vi "Planet_Meassurement.vi"(8 "error in (no error)":errorcluster, 11 "Conf":T1) -> (0 "error out":errorcluster)   [LabVIEW 2021]
uses:
  Typedefs/Stany.ctl
  Typedefs/Axis.ctl
  Typedefs/OrderAnalysis.ctl
  Typedefs/Start_End.ctl
  Typedefs/PropertiesOrderAnalysis.ctl
  Typedefs/FGV_TDMS.ctl
  Typedefs/GET_SET.ctl
  Typedefs/PropertyUserChange.ctl
  Typedefs/DataToUserInterface.ctl
  Typedefs/MeassurementMode.ctl
  Typedefs/PropertiesRead_TDM.ctl
  <vilib>/DAQmx/create/channels.llb/DAQmx Create Channel (AI-Voltage-Basic).vi
  <vilib>/DAQmx/read.llb/DAQmx Read (Analog 1D Wfm NChan NSamp).vi
  <vilib>/DAQmx/configure/timing.llb/DAQmx Timing (Sample Clock).vi
  Typedefs/Detected peaks.ctl
  Typedefs/All_Queues.ctl
  Typedefs/ConfCluster.ctl
  Typedefs/PlanetInfo.ctl
  Typedefs/AllDataToAnal.ctl
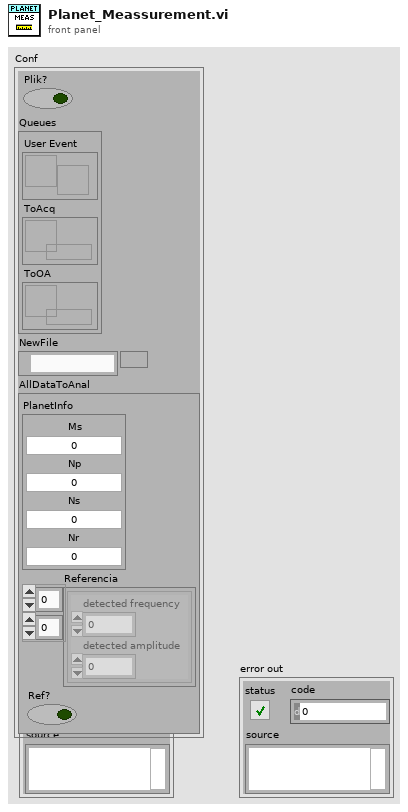
[diagram p1: front panel]
types:
  T1 = typedef "ConfCluster.ctl" = cluster{"Plik?":bool, "Queues":T2, "NewFile":path, "AllDataToAnal":T3}
  T2 = typedef "All_Queues.ctl" = cluster{"User Event":refnum<user-event>, "ToAcq":refnum<queue>, "ToOA":refnum<queue>}
  T3 = typedef "AllDataToAnal.ctl" = cluster{"PlanetInfo":T4, "Referencia":T5[][], "Ref?":bool}
  T4 = typedef "PlanetInfo.ctl" = cluster{"Ms":dbl, "Np":dbl, "Ns":dbl, "Nr":dbl}
  T5 = typedef "Detected peaks.ctl" = cluster{"detected frequency":dbl, "detected amplitude":dbl}
  T6 = typedef "PropertiesRead_TDM.ctl" = cluster{"Start/End":T7, "stop":bool, "file path":path, "OrderAnalysis":T8, "Meassurement Mode":T10}
  T7 = typedef "Start_End.ctl" = enum16{"Start", "End"}
  T8 = typedef "OrderAnalysis.ctl" = cluster{"dB on":bool, "window type":u32, "max order to analyze":dbl, "order resolution":dbl, "Axis":T9, "Sample rate":i64, "Save?":bool, "Multiple_Frequency":i32, "averaging mode":enum16{"No averaging", "Vector averaging", "RMS averaging", "Peak hold"}}
  T9 = typedef "Axis.ctl" = u16
  T10 = typedef "MeassurementMode.ctl" = cluster{"Sample mode":i32, "Terminal conf":i32, "Channels":tag}
  T11 = typedef "Stany.ctl" = enum16{"Idle", "Init", "Acq", "End"}
  T12 = typedef "PropertiesOrderAnalysis.ctl" = cluster{"Start/End":T7, "data":waveform(dbl)[], "OrderAnalysis":T8, "Tacho":waveform(dbl)[]}
  T13 = typedef "PropertyUserChange.ctl" = enum16{"Default", "Results", "Start", "Save", "CanalNames"}
  T14 = typedef "DataToUserInterface.ctl" = cluster{"Value":variant, "Property":T13}
  T15 = typedef "GET_SET.ctl" = enum16{"SET", "GET"}
  T16 = typedef "FGV_TDMS.ctl" = cluster{"Counter":i32, "Syg_GroupName":string, "Syg_ChannelNames":string[], "Tacho_GroupName":string, "Tacho_ChannelNames":string[]}
  T17 = enum16{"open", "open or create", "create or replace", "create", "open (read-only)"}
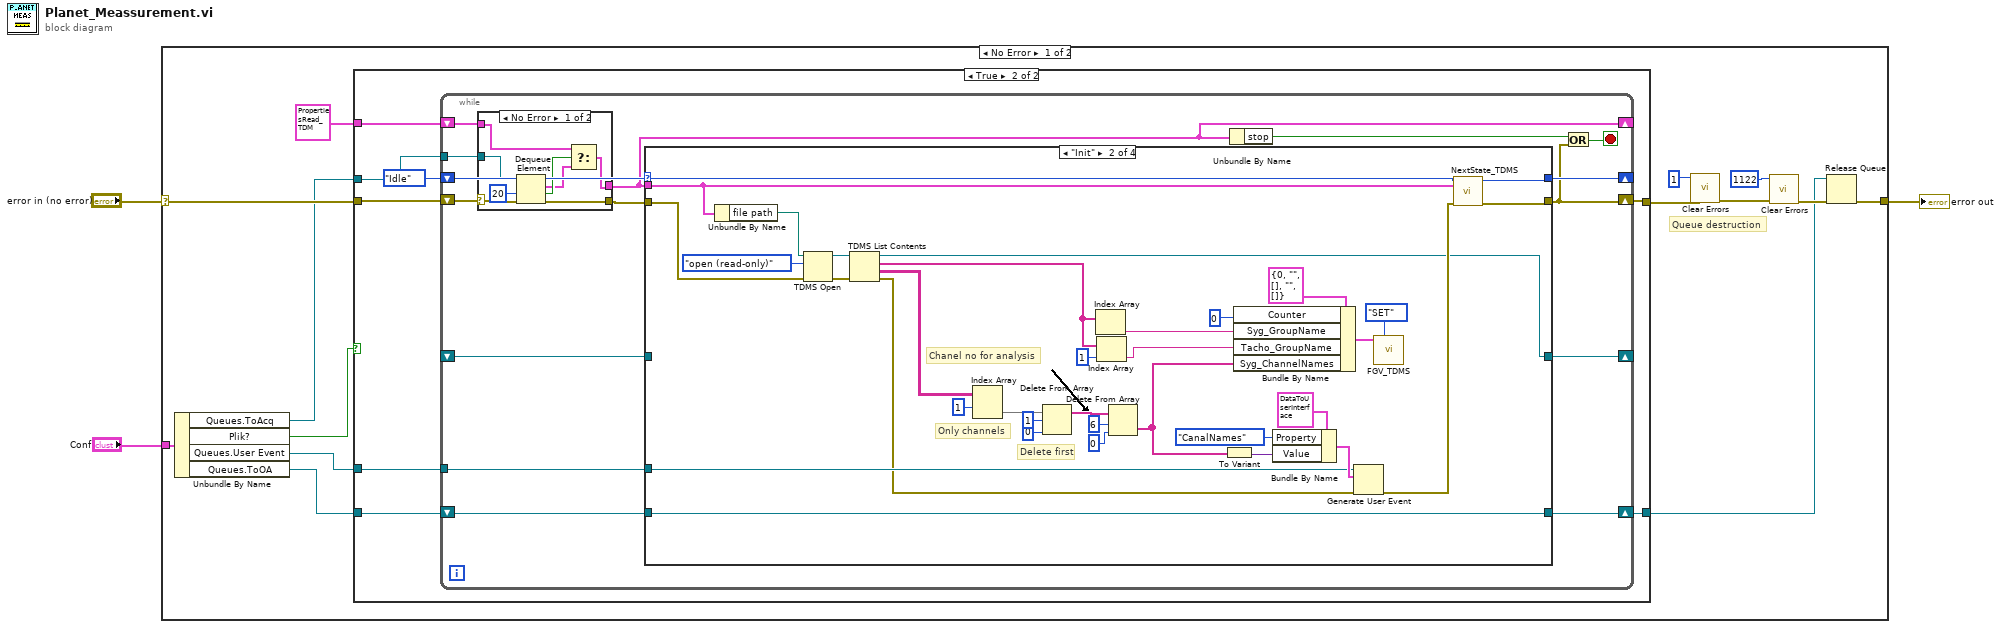
[diagram p0: block diagram]
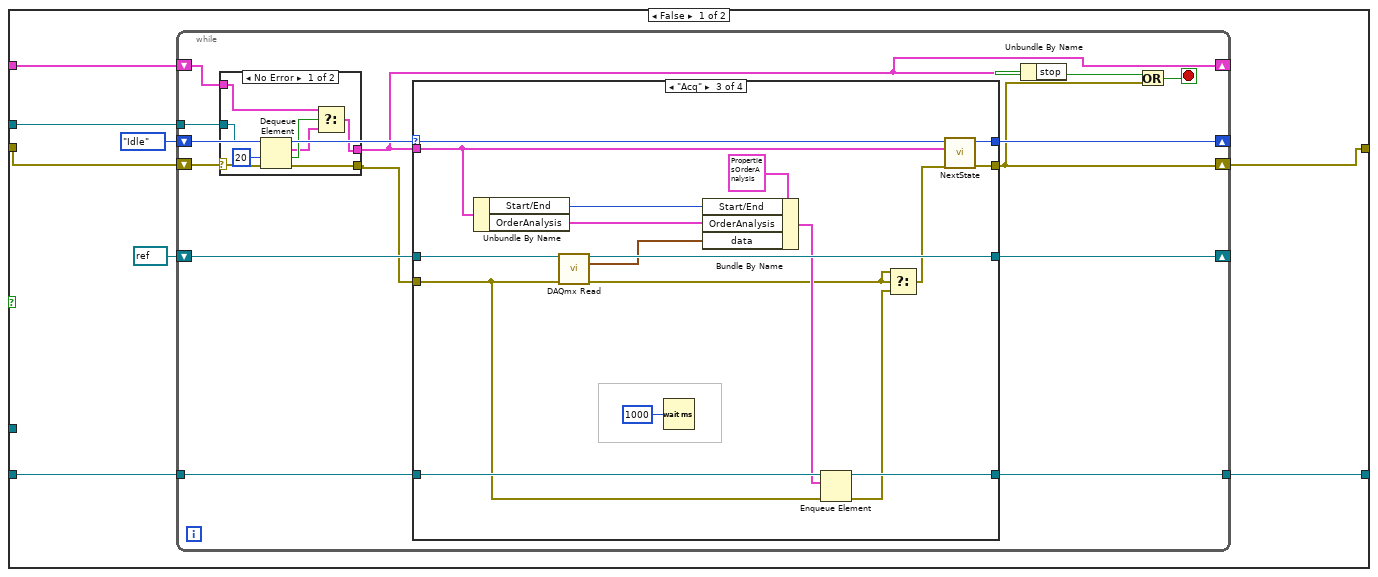
[diagram p2: hidden frame]
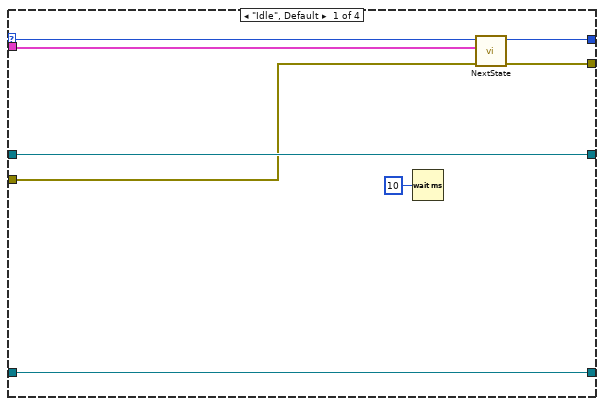
[diagram p4: hidden frame]
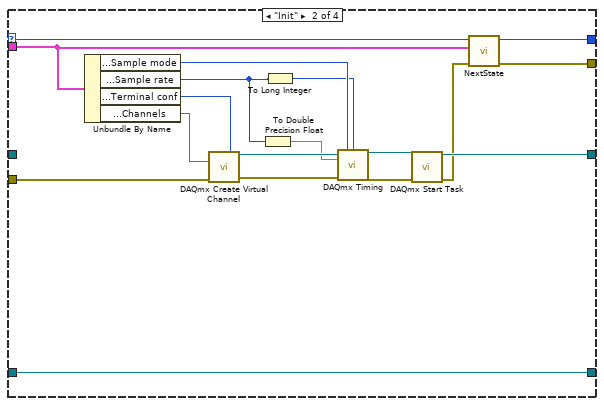
[diagram p5: hidden frame]
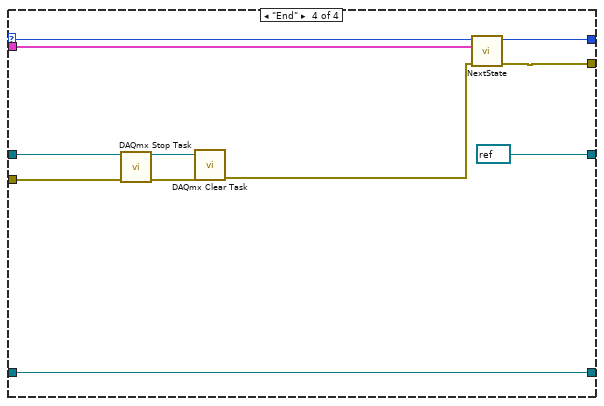
[diagram p6: hidden frame]
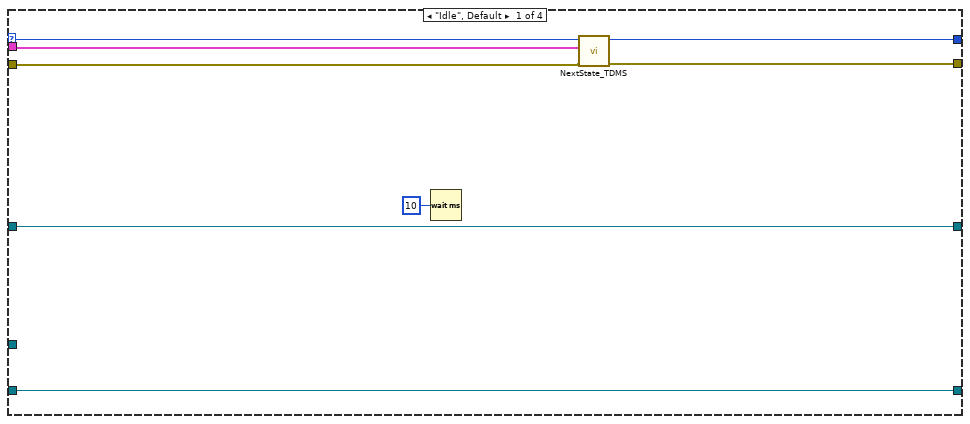
[diagram p8: hidden frame]
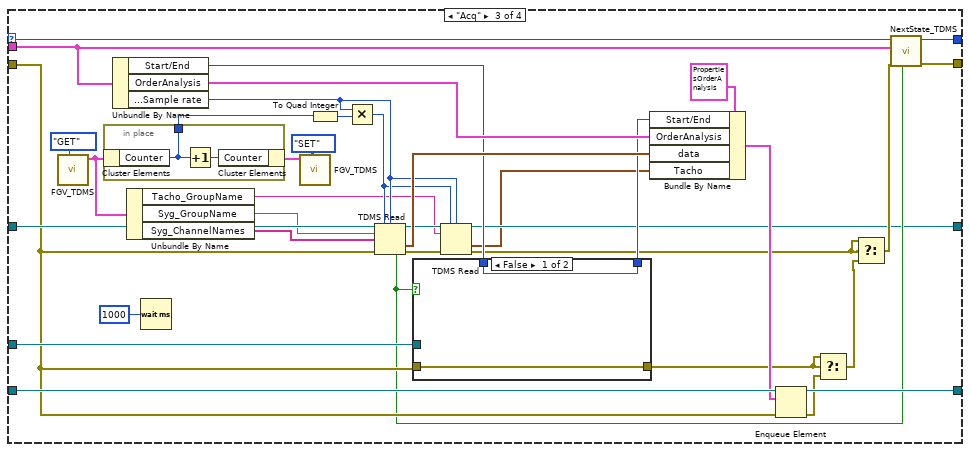
[diagram p9: hidden frame]
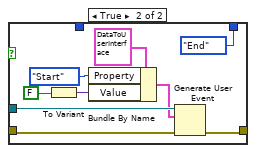
[diagram p10: hidden frame]
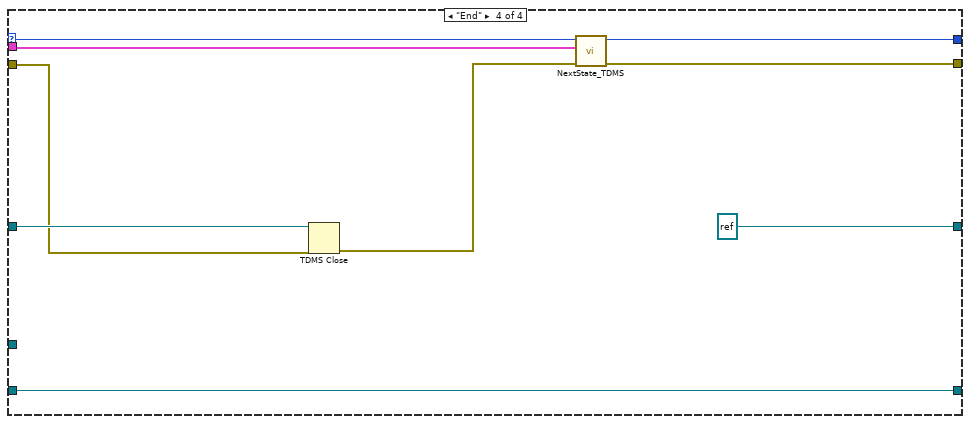
[diagram p11: hidden frame]
diagram:
  n1 = case shown="No Error" "error in (no error)" {
    selector: "error in (no error)" -> [w16 w240]
    tunnel: [w17 w240] -> w3
    tunnel: "Conf" -> [w11 _]
    frame No Error {
      # "Queue destruction"
      n2 = Unbundle By Name(w11) -> ("Queues.ToAcq"=w15:refnum<queue>, "Plik?"=w14:bool, "Queues.User Event"=w12:refnum<user-event>, "Queues.ToOA"=w13:refnum<queue>)
      n3 = case shown="True" w14 {
        tunnel: w16 -> [w24 w111]
        tunnel: T6 {"Start/End"=enum."End", "stop"=FALSE, "file path"=path "", "OrderAnalysis"={"dB on"=TRUE, "window type"=1, "max order to analyze"=32.0, "order resolution"=0.1, "Axis"=0, "Sample rate"=5000, "Save?"=FALSE, "Multiple_Frequency"=3, "averaging mode"=enum."No averaging"}, "Meassurement Mode"={"Sample mode"=10123, "Terminal conf"=12529, "Channels"=""}} -> [w22 w110]
        tunnel: [w20 w109] -> w5
        tunnel: w13 -> [w21 w108]
        tunnel: w12 -> [_ w107]
        tunnel: [w23 w106] -> w9
        tunnel: w15 -> [w18 w105]
        frame False {
          n4 = while {
            shift-right: [w38] -> _
            shift-left: refnum<k21> refnum ("task out") -> [w37]
            shift-right: [w36] -> _
            shift-left: Stany."Idle" -> [w39]
            shift-right: [w33] -> w23
            shift-left: w24 -> [w31]
            shift-right: [w29] -> _
            shift-left: w22 -> [w32]
            tunnel: w21 -> [w28]
            tunnel: [w27] -> w20
            tunnel: w18 -> [w26]
            stop <- w34 stop-if-true
            n5 = case shown="No Error" w31 {
              selector: w31 -> [w44 w49]
              tunnel: [w45 w49] -> w30
              tunnel: [w42 w48] -> w29
              tunnel: w32 -> [w41 w48]
              tunnel: w26 -> [w40 _]
              frame No Error {
                n6 = Dequeue Element(queue=w40, timeout in ms (-1)=20, error in (no error)=w44) -> (element=w43:T6, timed out?=w47:bool, error out=w45:errorcluster)  [unwired: 1 out]
                n7 = Select(t=w41, s=w47, f=w43) -> (s? t:f=w42:T6)
              }
              frame Error {
              }
            }
            n8 = case shown="\"Acq\"" w39 {
              selector: w39 -> [w54 w69 w89 w97]
              tunnel: [w57 w75 w92 refnum<k21> refnum ("task out")] -> w38
              tunnel: w37 -> [w57 _ w93 w104]
              tunnel: [w56 w66 w91 w99] -> w33
              tunnel: w30 -> [w52 w74 w86 w103]
              tunnel: w29 -> [w53 w65 w83 w96]
              tunnel: [w55 w68 w90 w98] -> w36
              tunnel: w28 -> [w50 w58 w87 w94]
              tunnel: [w50 w58 w85 w94] -> w27
              frame "Idle", Default {
                n9 = Wait (ms)(milliseconds to wait=u32 10) -> ()  [unwired: 1 out]
                n10 = call "NextState.vi"("error in (no error)"=w52, 10:w53, "Previous Step"=w54) -> ("error out"=w56:errorcluster, "Next Step"=w55:T11)  [unwired: 7 in]
              }
              frame "Init" {
                n11 = Unbundle By Name(w65) -> ("Meassurement Mode.Sample mode"=w62:i32, "OrderAnalysis.Sample rate"=w60:i64, "Meassurement Mode.Terminal conf"=w63:i32, "Meassurement Mode.Channels"=w61:tag)
                n12 = call-poly <vilib>:"DAQmx Create Virtual Channel.vi"("input terminal configuration"=w63, "physical channels"=w61, "error in"=w74) -> ("task out"=w73:refnum<k21>, "error out"=w70:errorcluster)  [unwired: 11 in]
                n13 = To Double Precision Float(number=w60) -> (double precision float=w64:dbl)
                n14 = To Long Integer(number=w60) -> (32bit integer=w59:i32)
                n15 = call-poly <vilib>:"DAQmx Timing.vi"("task/channels in"=w73, "sample mode"=w62, "samples per channel"=w59, "rate"=w64, "error in"=w70) -> ("task out"=w72:refnum<k21>, "error out"=w71:errorcluster)  [unwired: 9 in]
                n16 = call <vilib>:"DAQmx Start Task.vi"("task/channels in"=w72, "error in"=w71) -> ("task out"=w75:refnum<k21>, "error out"=w67:errorcluster)  [unwired: 12 in]
                n17 = call "NextState.vi"("error in (no error)"=w67, 10:w65, "Previous Step"=w69) -> ("error out"=w66:errorcluster, "Next Step"=w68:T11)  [unwired: 7 in]
              }
              frame "Acq" {
                n18 = Unbundle By Name(w83) -> ("Start/End"=w82:T7, "OrderAnalysis"=w81:T8)
                n19 = call-poly <vilib>:"DAQmx Read.vi"("task/channels in"=w93, "error in"=w86) -> ("task out"=w92:refnum<k21>, "data"=w76:waveform(dbl)[], "error out"=w79:errorcluster)  [unwired: 11 in]
                n20 = Wait (ms)(milliseconds to wait=u32 1000) -> ()  [unwired: 1 out]
                n21 = Bundle By Name(cluster=T12 {"Start/End"=enum."Start", "data"=[], "OrderAnalysis"={"dB on"=TRUE, "window type"=1, "max order to analyze"=32.0, "order resolution"=0.1, "Axis"=0, "Sample rate"=5000, "Save?"=FALSE, "Multiple_Frequency"=3, "averaging mode"=enum."No averaging"}, "Tacho"=[]}, "Start/End"=w82, "OrderAnalysis"=w81, "data"=w76) -> (w84:T12)
                n22 = Enqueue Element(queue=w87, element=w84, error in (no error)=w86) -> (queue out=w85:refnum<queue>, error out=w80:errorcluster)  [unwired: 1 in, 1 out]
                n23 = Select(t=w79, s=w79, f=w80) -> (s? t:f=w78:errorcluster)
                n24 = call "NextState.vi"("error in (no error)"=w78, 10:w83, "Previous Step"=w89) -> ("error out"=w91:errorcluster, "Next Step"=w90:T11)  [unwired: 7 in]
              }
              frame "End" {
                n25 = call <vilib>:"DAQmx Stop Task.vi"("task/channels in"=w104, "error in"=w103) -> ("task out"=w102:refnum<k21>, "error out"=w101:errorcluster)  [unwired: 12 in]
                n26 = call <vilib>:"DAQmx Clear Task.vi"("task in"=w102, "error in"=w101) -> ("error out"=w95:errorcluster)  [unwired: 13 in]
                n27 = call "NextState.vi"("error in (no error)"=w95, 10:w96, "Previous Step"=w97) -> ("error out"=w99:errorcluster, "Next Step"=w98:T11)  [unwired: 7 in]
              }
            }
            n28 = Unbundle By Name(w29) -> ("stop"=w35:bool)
            n29 = Or(x=w35, y=w33) -> (x .or. y?=w34:bool)
          }
        }
        frame True {
          n30 = while {
            shift-right: [w126] -> _
            shift-left: _ -> [w125]
            shift-right: [w124] -> _
            shift-left: Stany."Idle" -> [w127]
            shift-right: [w121] -> w106
            shift-left: w111 -> [w118]
            tunnel: w105 -> [w120]
            shift-right: [w116] -> _
            shift-left: w110 -> [w119]
            shift-right: [w115] -> w109
            shift-left: w108 -> [w114]
            tunnel: w107 -> [w113]
            stop <- w122 stop-if-true
            n31 = case shown="No Error" w118 {
              selector: w118 -> [w132 w137]
              tunnel: [w133 w137] -> w117
              tunnel: [w130 w136] -> w116
              tunnel: w120 -> [w129 _]
              tunnel: w119 -> [w128 w136]
              frame No Error {
                n32 = Dequeue Element(queue=w129, timeout in ms (-1)=20, error in (no error)=w132) -> (element=w131:T6, timed out?=w135:bool, error out=w133:errorcluster)  [unwired: 1 out]
                n33 = Select(t=w128, s=w135, f=w131) -> (s? t:f=w130:T6)
              }
              frame Error {
              }
            }
            n34 = case shown="\"Init\"" w127 {
              selector: w127 -> [w141 w175 w213 w237]
              tunnel: [w145 w146 w186 refnum<k34> refnum ("tdms file out")] -> w126
              tunnel: w125 -> [w145 _ w216 w239]
              tunnel: [w143 w177 w215 w235] -> w121
              tunnel: w117 -> [w140 w149 w196 w232]
              tunnel: w116 -> [w139 w174 w212 w234]
              tunnel: [w142 w176 w214 w236] -> w124
              tunnel: [w138 w172 w211 w233] -> w115
              tunnel: w114 -> [w138 w172 w210 w233]
              tunnel: w113 -> [_ w151 w197 _]
              frame "Idle", Default {
                n35 = Wait (ms)(milliseconds to wait=u32 10) -> ()  [unwired: 1 out]
                n36 = call "NextState_TDMS.vi"("error in (no error)"=w140, 10:w139, "Previous Step"=w141) -> ("error out"=w143:errorcluster, "Next Step"=w142:T11)  [unwired: 7 in]
              }
              frame "Init" {
                # "Chanel no for analysis"
                # "Only channels"
                # "Delete first"
                n37 = Unbundle By Name(w174) -> ("file path"=w173:path)
                n38 = TDMS Open(8:w149, 10:T17."open (read-only)" ("operation (0:open)"), 11:w173) -> (0:w180:errorcluster, 3:w179:refnum<k34>)  [unwired: 4 in]
                n39 = TDMS List Contents(4:w180, 7:w179) -> (0:w147:errorcluster, 1:w159:string[][], 2:w166:string[], 3:w146:refnum<k34>)  [unwired: 1 in]
                n40 = Index Array(array=w159, index (row)=1) -> (element=w162:string[])  [unwired: 1 in]
                n41 = Delete From Array(array=w162, length=1, index=0) -> (array with subset deleted=w158:string[])  [unwired: 1 out]
                n42 = Index Array(array=w166) -> (element=w167:string)  [unwired: 1 in]
                n43 = Index Array(array=w166, index=1) -> (element=w164:string)
                n44 = Delete From Array(array=w158, length=6, index=0) -> (deleted portion=w150:string[])  [unwired: 1 out]
                n45 = To Variant(anything=w150) -> (Variant=w152:variant)
                n46 = Bundle By Name(cluster=T16 {"Counter"=0, "Syg_GroupName"="", "Syg_ChannelNames"=[], "Tacho_GroupName"="", "Tacho_ChannelNames"=[]}, "Counter"=0, "Syg_GroupName"=w167, "Tacho_GroupName"=w164, "Syg_ChannelNames"=w150) -> (w169:T16)
                n47 = Bundle By Name(cluster=T14 {"Value"=variant, "Property"=enum."Default"} ("UserData"), "Property"=PropertyUserChange."CanalNames", "Value"=w152) -> (w154:T14)
                n48 = Generate User Event(user event=w151, event data cluster=w154, error in=w147) -> (error out=w148:errorcluster)  [unwired: 1 in, 1 out]
                n49 = call "FGV_TDMS.vi"("GET/SET"=GET_SET."SET", "Prop in"=w169) -> ()  [unwired: 9 in, 1 out]
                n50 = call "NextState_TDMS.vi"("error in (no error)"=w148, 10:w174, "Previous Step"=w175) -> ("error out"=w177:errorcluster, "Next Step"=w176:T11)  [unwired: 7 in]
              }
              frame "Acq" {
                n51 = call "FGV_TDMS.vi"("GET/SET"=GET_SET."GET") -> ("Prop out"=w201:T16)  [unwired: 10 in]
                n52 = in-place {
                  in-place-border: [w230] -> w202
                  n53 = in-place-cluster #1(w201) -> ("Counter"=w230:i32)
                  n54 = Increment(x=w230) -> (x+1=w229:i32)
                  n55 = in-place-cluster #1("Counter"=w229) -> (w203:T16)
                }
                n56 = Unbundle By Name(w212) -> ("Start/End"=w195:T7, "OrderAnalysis"=w207:T8, "OrderAnalysis.Sample rate"=w184:i64)
                n57 = Unbundle By Name(w201) -> ("Tacho_GroupName"=w182:string, "Syg_GroupName"=w200:string, "Syg_ChannelNames"=w199:string[])
                n58 = Wait (ms)(milliseconds to wait=u32 1000) -> ()  [unwired: 1 out]
                n59 = call "FGV_TDMS.vi"("GET/SET"=GET_SET."SET", "Prop in"=w203) -> ()  [unwired: 9 in, 1 out]
                n60 = To Quad Integer(1:w202) -> (0:w217:i64)
                n61 = Multiply(x=w184, y=w217) -> (x*y=w183:i64)
                n62 = TDMS Read(0:w216, 1:w183, 2:w184, 5:w200, 7:w199, 11:w196) -> (4:w188:refnum<k34>, 10:w208:waveform(dbl)[], 14:w189:bool, 15:w187:errorcluster)  [unwired: 2 in, 2 out]
                n63 = case shown="False" w189 {
                  tunnel: w197 -> [_ w228]
                  tunnel: w196 -> [w219 w227]
                  tunnel: [w219 w226] -> w193
                  tunnel: w195 -> [w218 _]
                  tunnel: [w218 Start_End."End" ("Start/End")] -> w194
                  frame False {
                  }
                  frame True {
                    n64 = To Variant(anything=FALSE) -> (Variant=w221:variant)
                    n65 = Bundle By Name(cluster=T14 {"Value"=variant, "Property"=enum."Default"} ("UserData"), "Property"=PropertyUserChange."Start", "Value"=w221) -> (w224:T14)
                    n66 = Generate User Event(user event=w228, event data cluster=w224, error in=w227) -> (error out=w226:errorcluster)  [unwired: 1 in, 1 out]
                  }
                }
                n67 = TDMS Read(0:w188, 1:w183, 2:w184, 5:w182, 11:w187) -> (4:w186:refnum<k34>, 10:w181:waveform(dbl)[], 15:w185:errorcluster)  [unwired: 3 in, 3 out]
                n68 = Bundle By Name(cluster=T12 {"Start/End"=enum."Start", "data"=[], "OrderAnalysis"={"dB on"=TRUE, "window type"=1, "max order to analyze"=32.0, "order resolution"=0.1, "Axis"=0, "Sample rate"=5000, "Save?"=FALSE, "Multiple_Frequency"=3, "averaging mode"=enum."No averaging"}, "Tacho"=[]}, "Start/End"=w194, "OrderAnalysis"=w207, "data"=w208, "Tacho"=w181) -> (w206:T12)
                n69 = Enqueue Element(queue=w210, element=w206, error in (no error)=w196) -> (queue out=w211:refnum<queue>, error out=w192:errorcluster)  [unwired: 1 in, 1 out]
                n70 = Select(t=w193, s=w193, f=w192) -> (s? t:f=w191:errorcluster)
                n71 = Select(t=w185, s=w185, f=w191) -> (s? t:f=w190:errorcluster)
                n72 = call "NextState_TDMS.vi"("end of file?"=w189, "error in (no error)"=w190, 10:w212, "Previous Step"=w213) -> ("error out"=w215:errorcluster, "Next Step"=w214:T11)  [unwired: 6 in]
              }
              frame "End" {
                n73 = TDMS Close(8:w232, 11:w239) -> (0:w231:errorcluster)  [unwired: 1 out]
                n74 = call "NextState_TDMS.vi"("error in (no error)"=w231, 10:w234, "Previous Step"=w237) -> ("error out"=w235:errorcluster, "Next Step"=w236:T11)  [unwired: 7 in]
              }
            }
            n75 = Unbundle By Name(w116) -> ("stop"=w123:bool)
            n76 = Or(x=w123, y=w121) -> (x .or. y?=w122:bool)
          }
        }
      }
      n77 = call <vilib>:"Clear Errors.vi"("error in (no error)"=w9, "specific error code to clear (0: all)"=1) -> ("error out"=w7:errorcluster)  [unwired: 4 in, 1 out]
      n78 = call <vilib>:"Clear Errors.vi"("error in (no error)"=w7, "specific error code to clear (0: all)"=1122) -> ("error out"=w10:errorcluster)  [unwired: 4 in, 1 out]
      n79 = Release Queue(queue=w5, error in (no error)=w10) -> (error out=w17:errorcluster)  [unwired: 1 in, 2 out]
    }
    frame Error {
    }
  }
  "error out" <- w3
